vi "CRYGet Calibration 2D From Signal Type.vi"(10 "I/O Calibration 2D":T1[](array[typedef]) {"Sens Curve"."Z data" items=["dB", "Lin"]; "Sens Curve"."X data" items=["dB", "Lin"]; "Sens Curve"."Y data" items=["dB", "Lin"]; "Sens Curve"."Z dB ref" format="%.1f"; "Sens Curve"."Z axis" items=["Log", "Lin"]; "Sens Curve"."X dB ref" format="%.1f"; "Sens Curve"."X axis" items=["Log", "Lin"]; "Sens Curve"."Y axis" items=["Log", "Lin"]; "Sens Curve"."Y dB ref" format="%.1f"; "Sens Curve"."Curve"."z" format="%.2f"; "Sens Curve"."Curve"."y" format="%.2f"; "Sens Curve"."Curve"."x" format="%.2f"; "EQ Curve"."Z data" items=["dB", "Lin"]; "EQ Curve"."X data" items=["dB", "Lin"]; "EQ Curve"."Y data" items=["dB", "Lin"]; "EQ Curve"."Z dB ref" format="%.1f"; "EQ Curve"."Z axis" items=["Log", "Lin"]; "EQ Curve"."X dB ref" format="%.1f"; "EQ Curve"."X axis" items=["Log", "Lin"]; "EQ Curve"."Y axis" items=["Log", "Lin"]; "EQ Curve"."Y dB ref" format="%.1f"; "EQ Curve"."Curve"."z" format="%.2f"; "EQ Curve"."Curve"."y" format="%.2f"; "EQ Curve"."Curve"."x" format="%.2f"; "Corr Curve"."Z data" items=["dB", "Lin"]; "Corr Curve"."X data" items=["dB", "Lin"]; "Corr Curve"."Y data" items=["dB", "Lin"]; "Corr Curve"."Z dB ref" format="%.1f"; "Corr Curve"."Z axis" items=["Log", "Lin"]; "Corr Curve"."X dB ref" format="%.1f"; "Corr Curve"."X axis" items=["Log", "Lin"]; "Corr Curve"."Y axis" items=["Log", "Lin"]; "Corr Curve"."Y dB ref" format="%.1f"; "Corr Curve"."Curve"."z" format="%.2f"; "Corr Curve"."Curve"."y" format="%.2f"; "Corr Curve"."Curve"."x" format="%.2f"; "Calibration"."EQ Step size" items=["R10", "R20", "R40", "R80", "User"]; "Calibration"."Corr Step size" items=["R10", "R20", "R40", "R80", "User"]}, 11 "Signal Type Name In":string) -> (2 "equal Index Out":i32, 3 "Channel Name Out":string)   [LabVIEW 2013]
uses:
  Typedef Control/CRYCalibration 2DCluster.ctl
  Typedef Control/CRYCalibration Cluster.ctl
  Typedef Control/CRYData Cluster.ctl
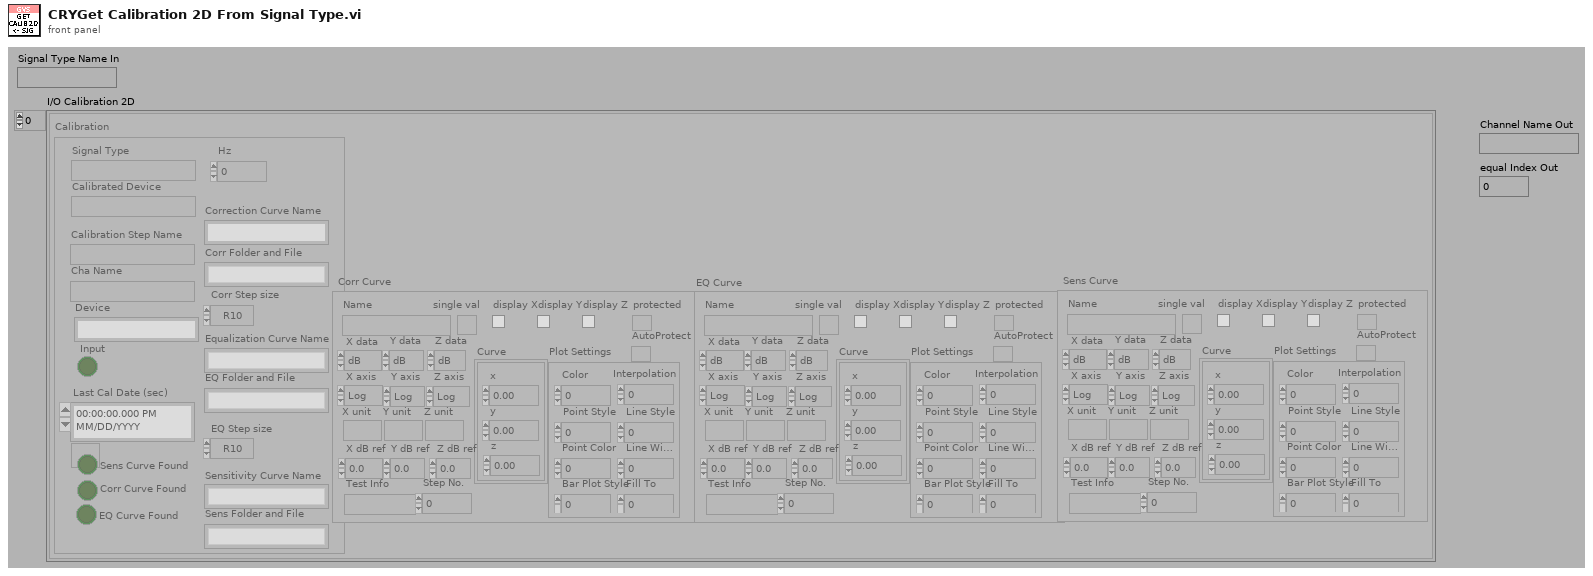
[diagram p1: front panel]
types:
  T1 = typedef "CRYCalibration 2DCluster.ctl" = cluster{"Calibration":T2, "Corr Curve":T3, "EQ Curve":T3, "Sens Curve":T3}
  T2 = typedef "CRYCalibration Cluster.ctl" = cluster{"Calibration Step Name":string, "Device":string, "Correction Curve Name":string, "Equalization Curve Name":string, "Sensitivity Curve Name":string, "Corr Folder and File":string, "EQ Folder and File":string, "Sens Folder and File":string, "Corr Step size":u16, "EQ Step size":u16, "Input":bool, "Last Cal Date (sec)":timestamp, "Cha Name":string, "Corr Curve Found":bool, "EQ Curve Found":bool, "Sens Curve Found":bool, "Signal Type":string, "Calibrated Device":string, "Hz":u32}
  T3 = typedef "CRYData Cluster.ctl" = cluster{"Name":string, "Curve":cluster{"x":dbl, "y":dbl, "z":dbl}[], "X data":u16, "Y data":u16, "Z data":u16, "X axis":u16, "Y axis":u16, "Z axis":u16, "X unit":string, "Y unit":string, "Z unit":string, "X dB ref":dbl, "Y dB ref":dbl, "Z dB ref":dbl, "single val":bool, "protected":bool, "display X":bool, "display Y":bool, "display Z":bool, "Test Info":string, "Step No.":i32, "Plot Settings":cluster{"Color":u32, "Interpolation":u8, "Point Style":u8, "Line Style":u8, "Point Color":u32, "Line Width":u8, "Bar Plot Style":u8, "Fill To":i16}, "AutoProtect":bool}
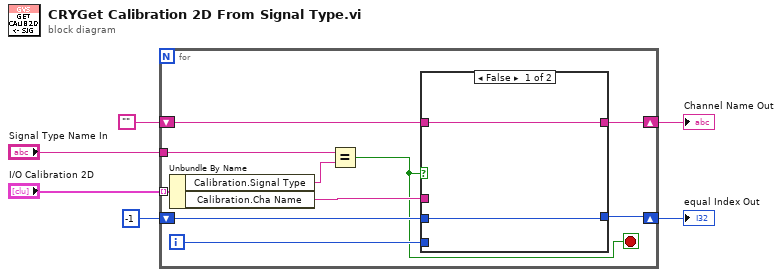
[diagram p0: block diagram]
diagram:
  n1 = for {
    tunnel: "I/O Calibration 2D" -> [w16] mode=indexing
    tunnel: "Signal Type Name In" -> [w12]
    shift-right: [w14] -> w3
    shift-left: "" ("Signal Type") -> [w15]
    shift-right: [w9] -> w4
    shift-left: -1 -> [w8]
    i -> [w10]
    stop <- w7 stop-if-true
    n2 = Unbundle By Name(w16) -> ("Calibration.Signal Type"=w13:string, "Calibration.Cha Name"=w11:string)
    n3 = Equal?(x=w12, y=w13) -> (x = y?=w7:bool)
    n4 = case shown="False" w7 {
      tunnel: w15 -> [w18 _]
      tunnel: [w18 w19] -> w14
      tunnel: w11 -> [_ w19]
      tunnel: w10 -> [_ w20]
      tunnel: [w17 w20] -> w9
      tunnel: w8 -> [w17 _]
      frame False {
      }
      frame True {
      }
    }
  }
  "equal Index Out" <- w4
  "Channel Name Out" <- w3
